vi "EditUser-Window.vi"(7 "Login-UI.lvlib:PwdMgr.lvclass":refnum<class "PwdMgr.lvclass">, 8 "error in":errorcluster, 9 "权  限":T1, 10 "密  码":string, 11 "用户名":string) -> (0 "error out":errorcluster)   [LabVIEW 2020, in "Login-UI.lvlib"]
uses:
  Login-UI.lvlib
  _Typedef/User-Role.ctl
  PwdMgr/PwdMgr.lvclass
  _Typedef/User-Info.ctl
panel:
  in  "Exit":bool
  in  "Save":bool
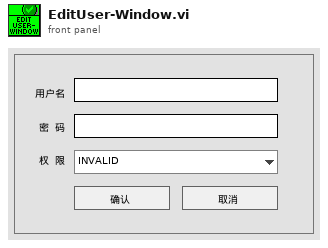
[diagram p1: front panel]
types:
  T1 = typedef "Login-UI.lvlib/User-Role.ctl" = enum16{"INVALID", "Operator", "Engineer", "Admin", "Anonymous"}
  T2 = enum32{"Invalid", "Standard", "Closed", "Hidden", "Minimized", "Maximized"}
  T3 = enum32{"invalid app kind", "Development System", "Run Time System", "Student Edition", "Embedded LabVIEW", "Evaluation", "Custom"}
  T4 = typedef "Login-UI.lvlib/User-Info.ctl" = cluster{"UserName":string, "Password":string, "Role":T1}
  T5 = cluster{"Core":cluster{"Current VI Reference":refnum<vi>, "Close Panel on Exit?":bool}, "Your Boolean data":bool, "Your string data":string, "Cluster":T4}
  T6 = typedef "eventvkey.ctl" = enum16{"ASCII", "Enter", "Return", "Shift", "Ctrl", "Alt", "Cmd", "Opt", "Caps", "NumLock", "Clear", "Break", "Up", "Down", "Left", "Right", "Insert", "Delete", "Home", "End", "PageUp", "PageDown", "Escape", "Help", "Pause", "ScrollLock", "F1", "F2", "F3", "F4", "F5", "F6", "F7", "F8", "F9", "F10", "F11", "F12", "F13", "F14", "F15", "F16", "F17", "F18", "F19", "F20", "F21", "F22", "F23", "F24", "Play", "VolumeUp", "VolumeDown", "Mute", "Two Byte Char"}
  T7 = cluster{"Current VI Reference":refnum<vi>, "Close Panel on Exit?":bool}
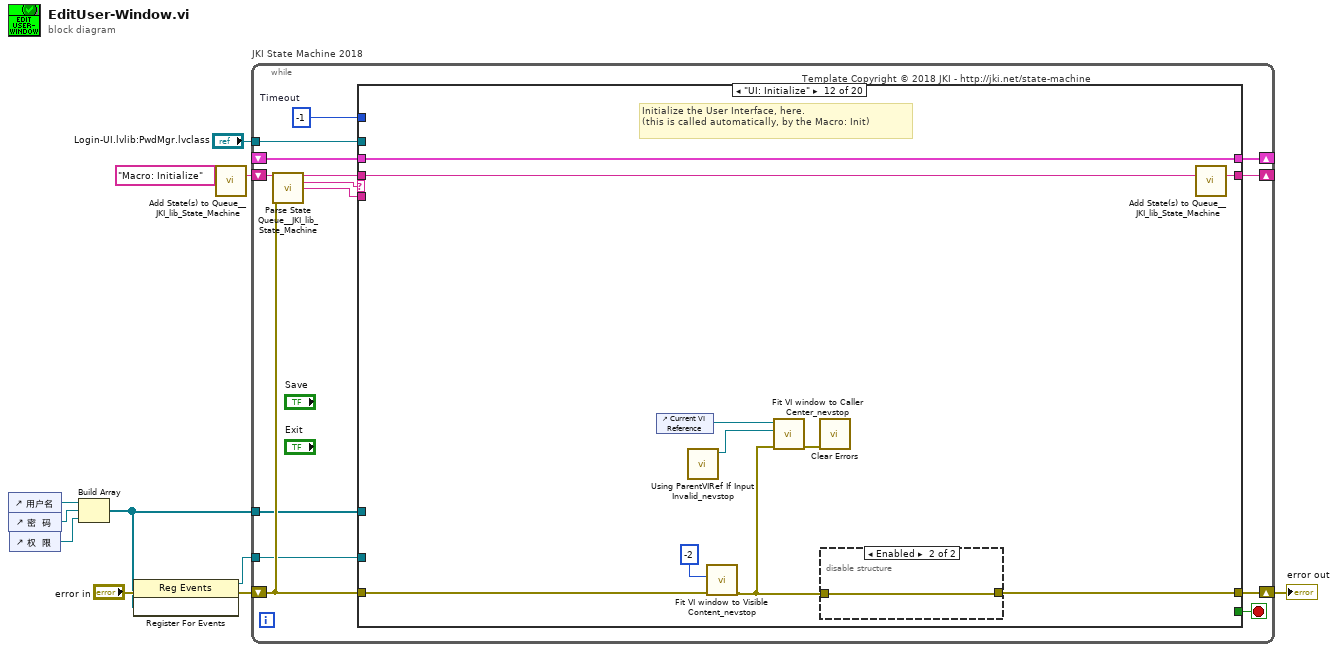
[diagram p0: block diagram]
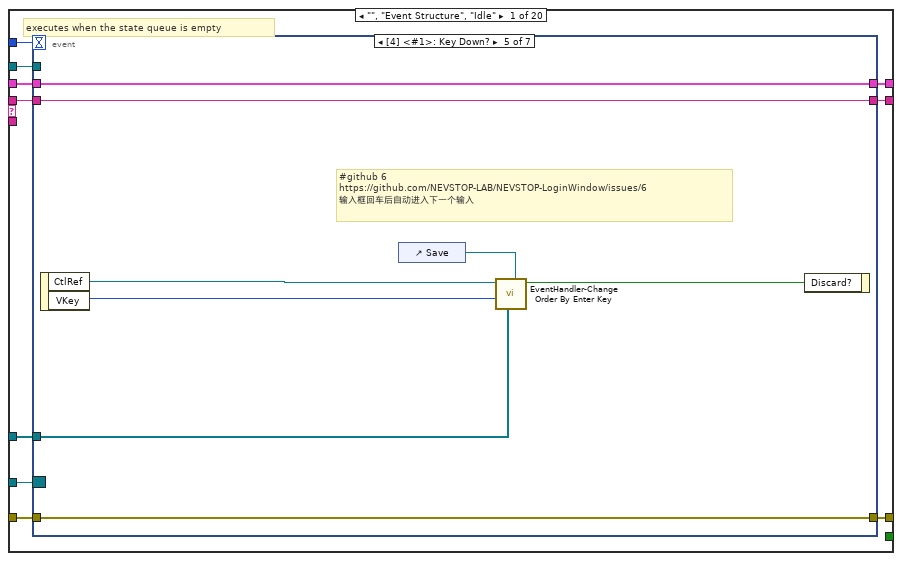
[diagram p2: hidden frame]
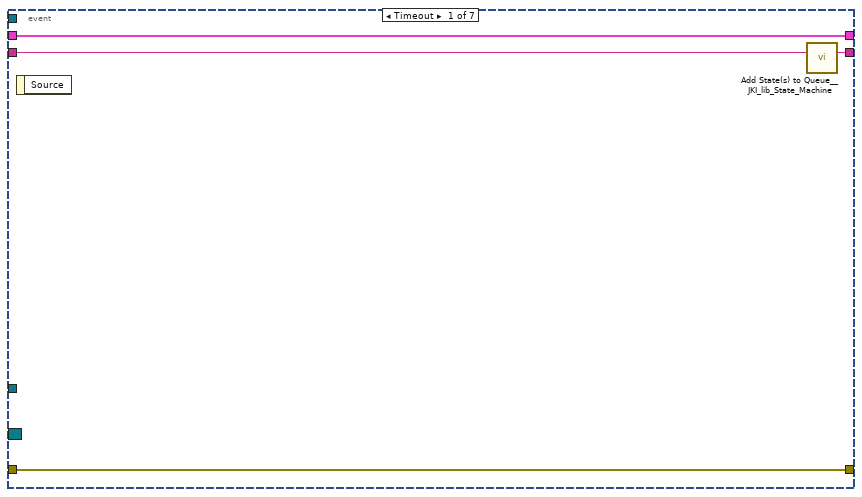
[diagram p3: hidden frame]
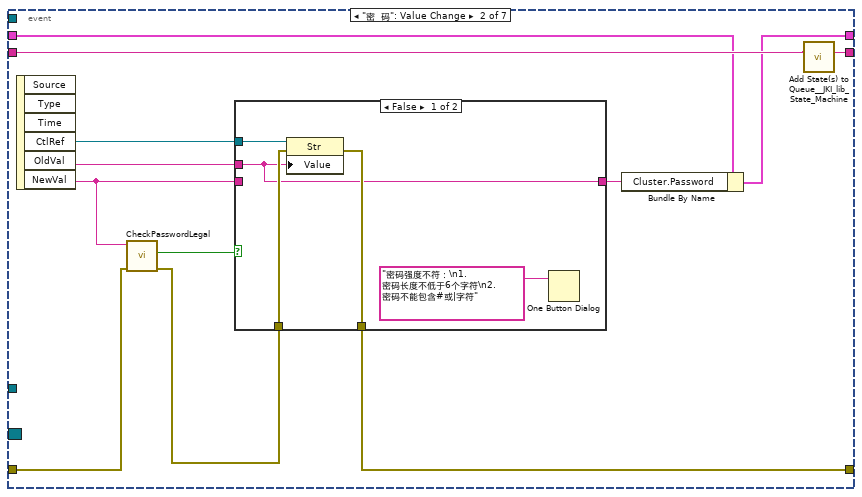
[diagram p4: hidden frame]
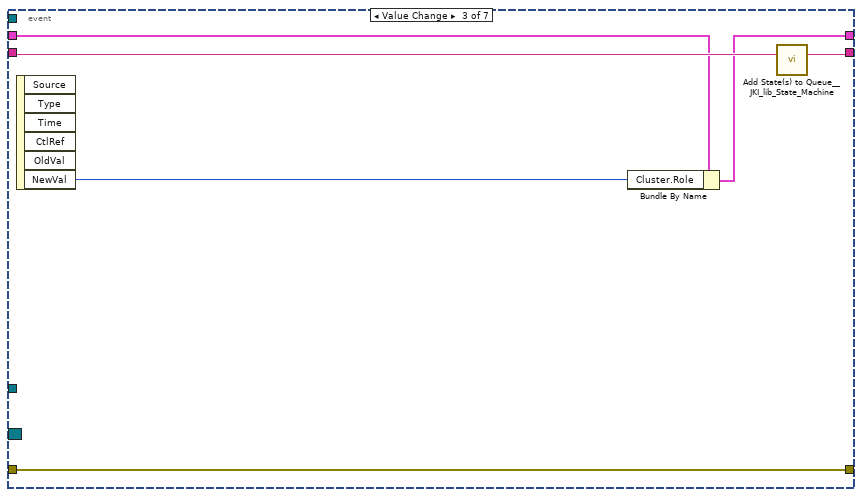
[diagram p6: hidden frame]
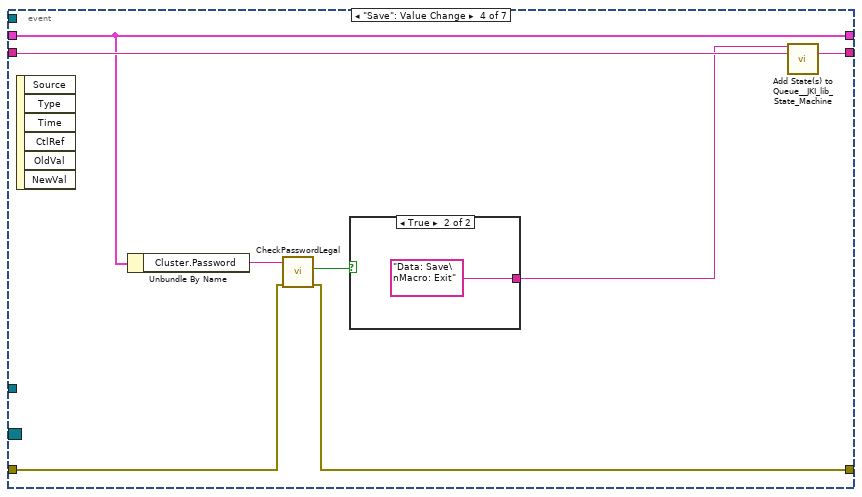
[diagram p7: hidden frame]
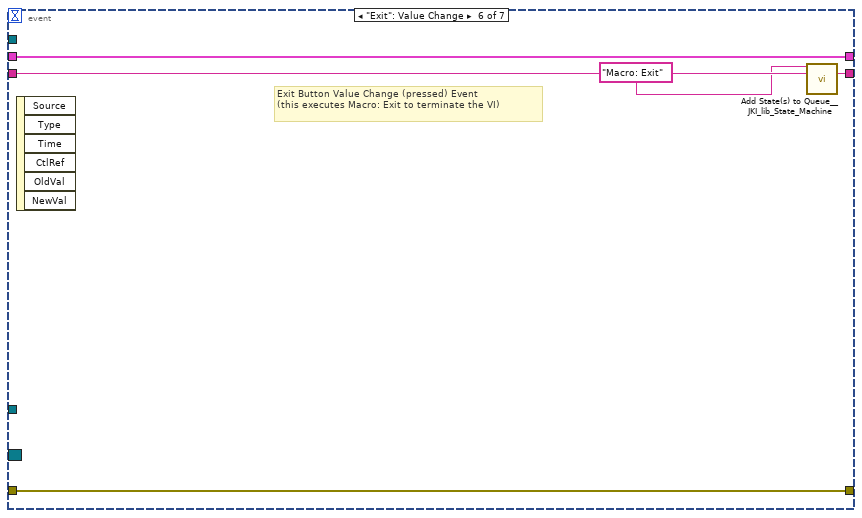
[diagram p9: hidden frame]
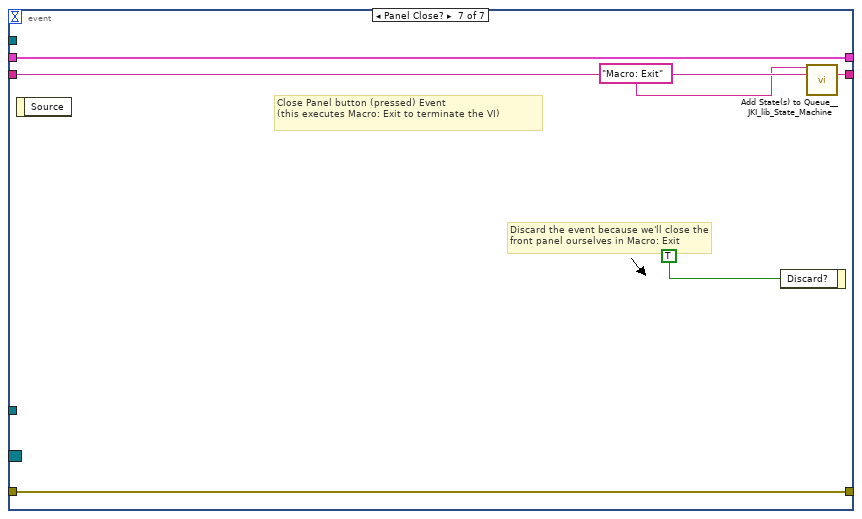
[diagram p10: hidden frame]
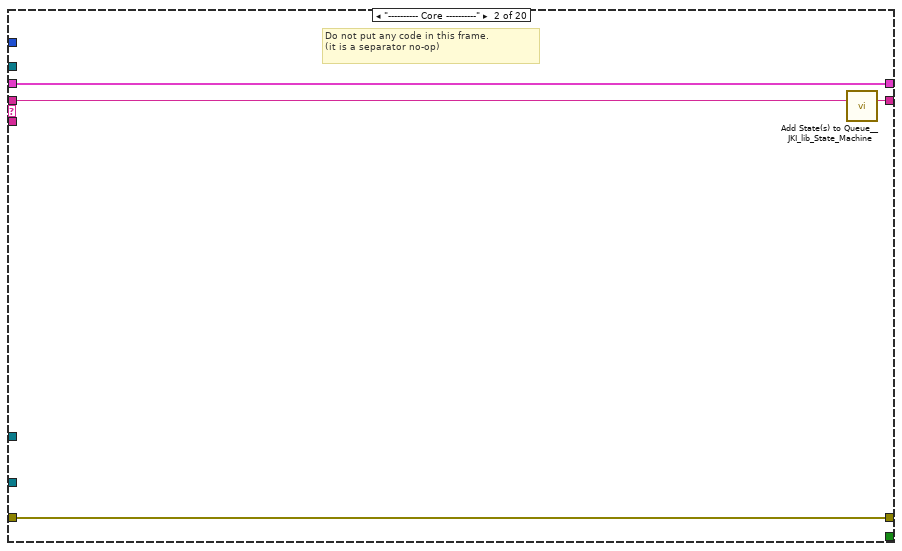
[diagram p11: hidden frame]
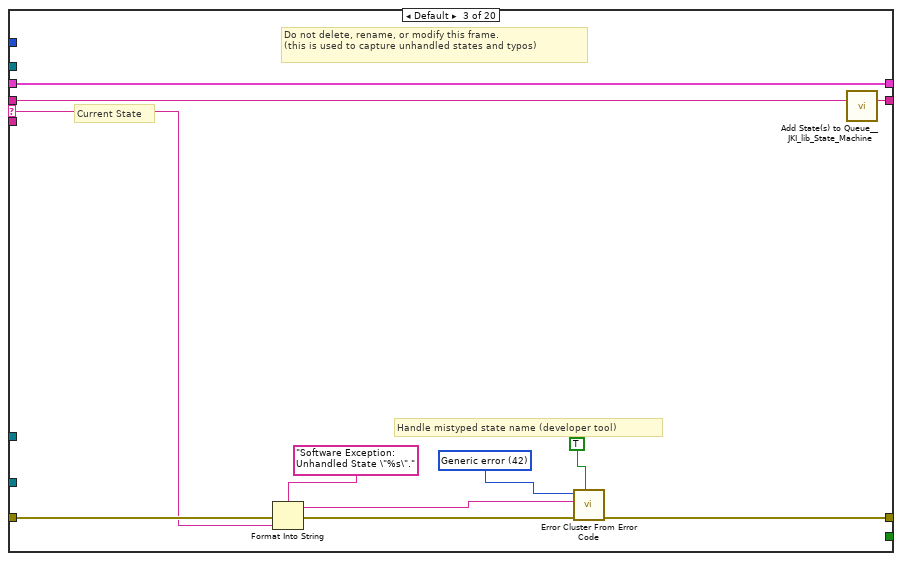
[diagram p12: hidden frame]
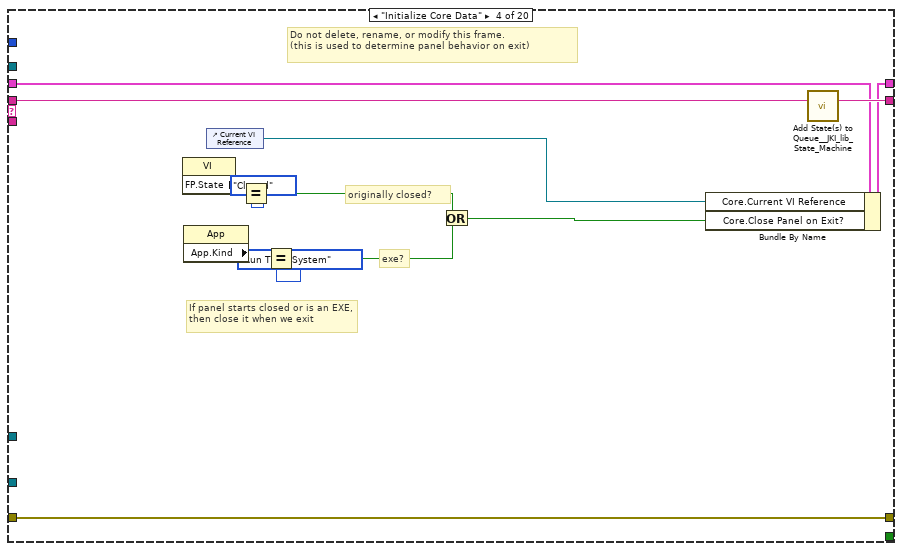
[diagram p13: hidden frame]
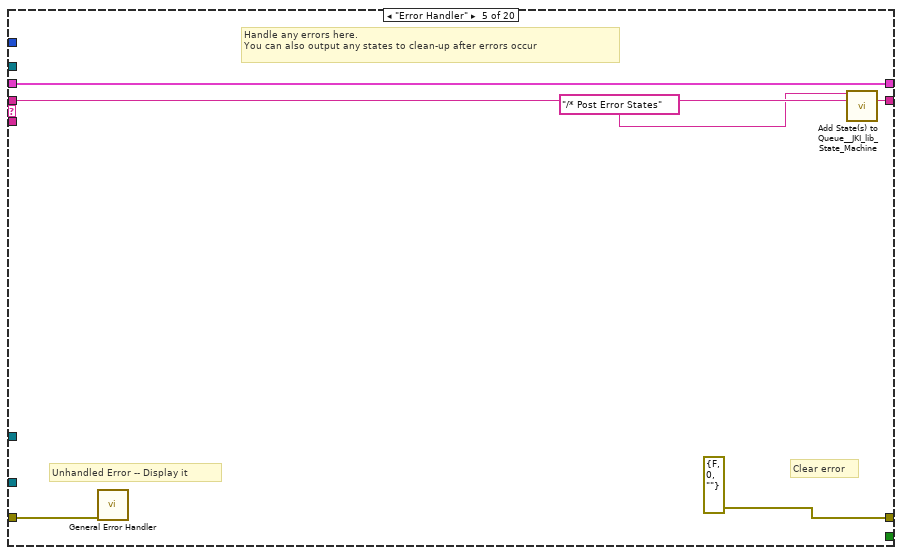
[diagram p14: hidden frame]
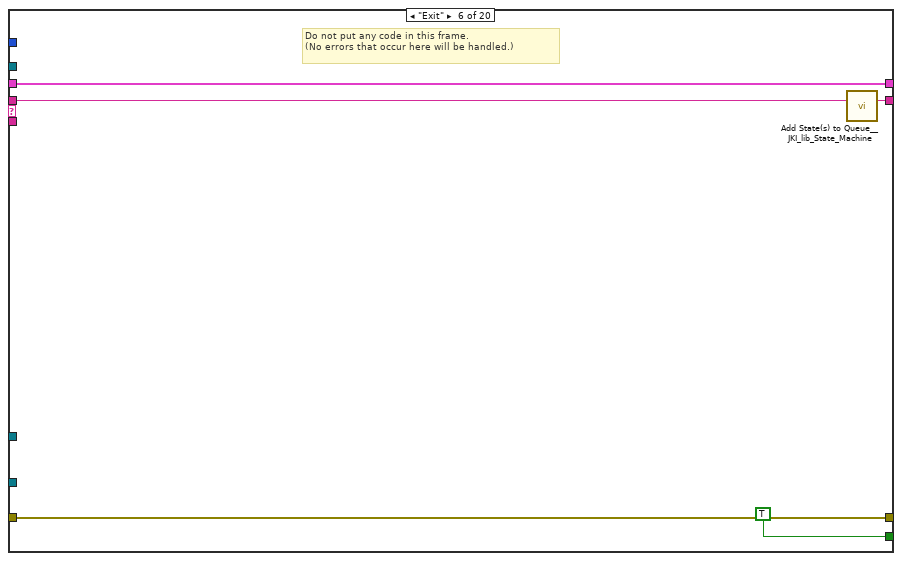
[diagram p15: hidden frame]
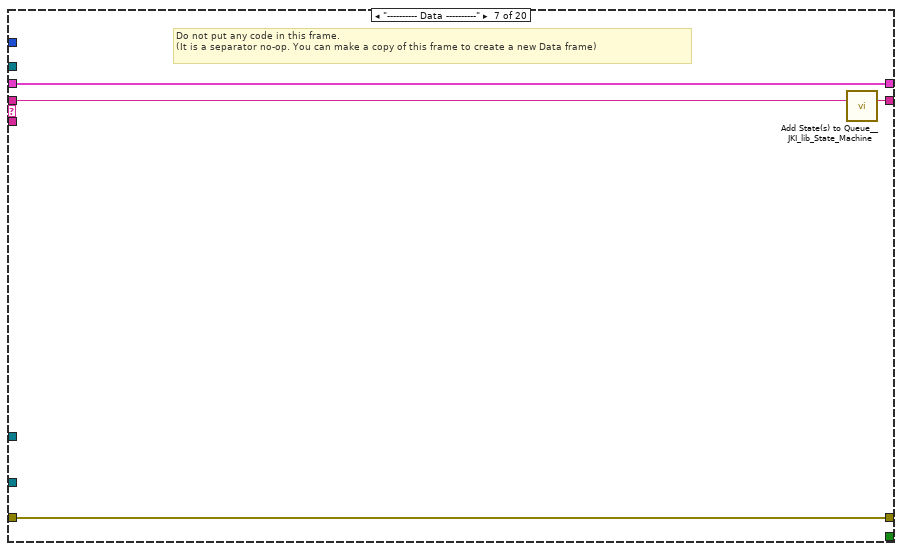
[diagram p16: hidden frame]
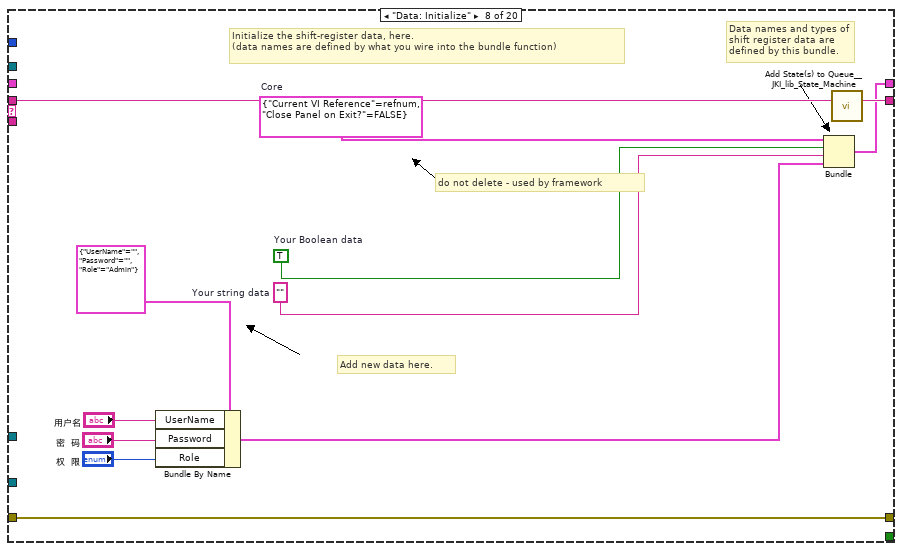
[diagram p17: hidden frame]
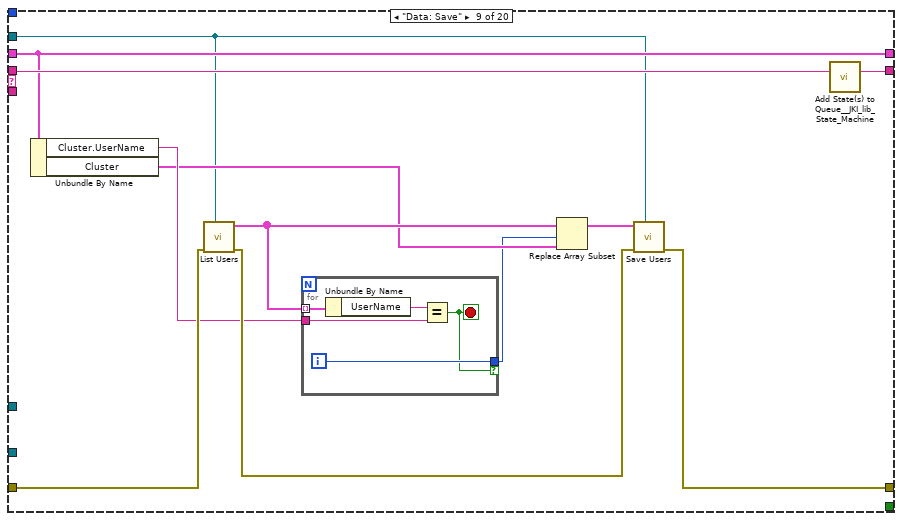
[diagram p18: hidden frame]
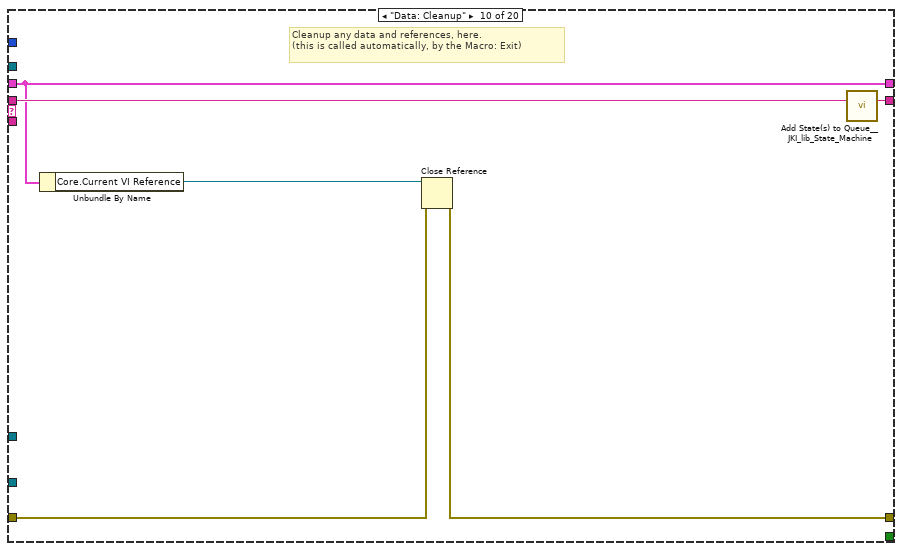
[diagram p19: hidden frame]
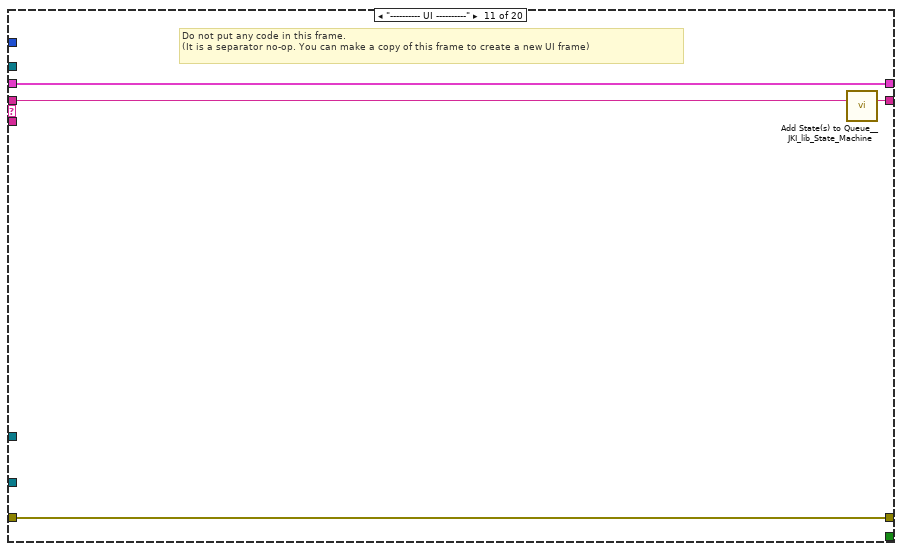
[diagram p20: hidden frame]
diagram:
  n1 = control-ref of="用户名"() -> (w6:refnum<vi>)
  n2 = control-ref of="密  码"() -> (w5:refnum<vi>)
  n3 = control-ref of="权  限"() -> (w4:refnum<vi>)
  n4 = Build Array(w6, w5, w4) -> (w2:refnum<vi>[])
  n5 = register-events(error in="error in", w2) -> (reference out=w3:refnum<event-registration>, error out=w7:errorcluster)  [unwired: 1 in]
  n6 = call <vilib>:"Add State(s) to Queue__JKI_lib_State_Machine.vi"("State(s) in (\"\")"="Macro: Initialize") -> ("States Out"=w11:string)  [unwired: 14 in]
  n7 = while "JKI State Machine 2018" {
    shift-right: [w18] -> _
    shift-left: _ -> [w17]
    shift-right: [w21] -> w8
    shift-left: w7 -> [w15]
    shift-right: [w20] -> _
    shift-left: w11 -> [w22]
    tunnel: w3 -> [w14]
    tunnel: w2 -> [w13]
    tunnel: "Login-UI.lvlib:PwdMgr.lvclass" -> [w12]
    stop <- w19 stop-if-true
    w16 = -1  # Timeout
    # "Template Copyright © 2018 JKI - http://jki.net/state-machine"
    n8 = call <vilib>:"Parse State Queue__JKI_lib_State_Machine.vi"("State Queue"=w22, "Error In (no error)"=w15) -> ("Remaining States"=w24:string, "Current State"=w25:string, "Arguments"=w23:string)  [unwired: 11 in]
    n9 = case shown="\"UI: Initialize\"" w25 {
      selector: w25 -> [_ _ w97 _ _ _ _ _ _ _ _ _ _ _ _ _ _ _ _ _]
      tunnel: w24 -> [w35 w96 w101 w120 w126 w131 w135 w147 w158 w170 w174 w184 w193 w204 w273 w278 w288 w292 w296 w300]
      tunnel: w23 -> [_ _ _ _ _ _ _ _ _ _ _ _ w188 w198 _ _ _ _ _ _]
      tunnel: w17 -> [w34 w93 w99 w113 w123 w129 w132 _ w157 w165 w171 w182 w191 w200 w270 w275 w285 w289 w293 w297]
      tunnel: [w33 w94 w103 w117 errorcluster {"status"=FALSE, "code"=0, "source"=""} ("error out") w128 w133 w144 w155 w166 w172 w179 w189 w201 w271 w276 w286 w290 w294 w298] -> w21
      tunnel: w15 -> [w32 w94 w102 w117 w122 w128 w133 w144 w156 w167 w172 w180 w190 w202 w271 w276 w286 w290 w294 w298]
      tunnel: [w29 w95 w100 w119 w125 w130 w134 w146 w159 w169 w173 w183 w192 w203 w272 w277 w287 w291 w295 w299] -> w20
      tunnel: [_ _ _ _ _ TRUE _ _ _ _ _ _ _ _ _ _ _ _ _ _] -> w19
      tunnel: [w31 w93 w99 w118 w123 w129 w132 w145 w157 w165 w171 w182 w191 w200 w270 w275 w285 w289 w293 w297] -> w18
      tunnel: w16 -> [w30 _ _ _ _ _ _ _ _ _ _ _ _ _ _ _ _ _ _ _]
      tunnel: w14 -> [w28 _ _ _ _ _ _ _ _ _ _ _ _ _ _ _ _ _ _ _]
      tunnel: w13 -> [w27 _ _ _ _ _ _ _ _ _ _ _ _ _ _ _ _ _ _ _]
      tunnel: w12 -> [w26 _ _ _ _ _ _ _ w148 _ _ _ _ _ _ _ _ _ _ _]
      frame "", "Event Structure", "Idle" {
        # "executes when the state queue is empty"
        n10 = event shown="[4] <#1>: Key Down?" {
          selector: w28 -> [_ _ _ _ _ _ _]
          dyn-events: _ -> [_ _ _ _ _ _ _]
          timeout: w30 -> [_ _ _ _ _ _ _]
          tunnel: w35 -> [w39 w47 w62 w71 w75 w86 w92]
          tunnel: [w38 w48 w63 w72 w75 w85 w91] -> w29
          tunnel: w34 -> [w36 w42 w61 w69 w76 w83 w89]
          tunnel: [w37 w49 w64 w65 w81 w84 w90] -> w33
          tunnel: w32 -> [w37 w45 w64 w66 w81 w84 w90]
          tunnel: [w36 w40 w60 w69 w76 w83 w89] -> w31
          tunnel: w27 -> [_ _ _ _ w78 _ _]
          tunnel: w26 -> [_ _ _ _ _ _ _]
          event Timeout {
            n11 = event-data() -> ()  [unwired: 1 in, 1 out]
            n12 = call <vilib>:"Add State(s) to Queue__JKI_lib_State_Machine.vi"("State(s) in (\"\")"=w39) -> ("States Out"=w38:string)  [unwired: 14 in]
          }
          event "密  码": Value Change {
            n13 = event-data() -> ("CtlRef"=w50:refnum<vi>, "OldVal"=w51:string, "NewVal"=w46:string)  [unwired: 1 in, 3 out]
            n14 = call "CheckPasswordLegal.vi"("error in (no error)"=w45, "Password"=w46) -> ("error out"=w44:errorcluster, "legal?"=w43:bool)  [unwired: 8 in]
            n15 = case shown="False" w43 {
              tunnel: w51 -> [w52 _]
              tunnel: w46 -> [_ w57]
              tunnel: [w55 w58] -> w49
              tunnel: w50 -> [w54 _]
              tunnel: w44 -> [w53 w58]
              tunnel: [w52 w57] -> w41
              frame False {
                n16 = property class="Str"(reference=w54, error in=w53, "Value"=w52) -> (error out=w55:errorcluster)  [unwired: 1 out]
                n17 = One Button Dialog(message="密码强度不符：\n1.密码长度不低于6个字符\n2. 密码不能包含#或|字符") -> ()  [unwired: 1 in, 1 out]
              }
              frame True {
              }
            }
            n18 = Bundle By Name(cluster=w42, "Cluster.Password"=w41) -> (w40:T5)
            n19 = call <vilib>:"Add State(s) to Queue__JKI_lib_State_Machine.vi"("State(s) in (\"\")"=w47) -> ("States Out"=w48:string)  [unwired: 14 in]
          }
          event Value Change {
            n20 = event-data() -> ("NewVal"=w59:T1)  [unwired: 1 in, 5 out]
            n21 = Bundle By Name(cluster=w61, "Cluster.Role"=w59) -> (w60:T5)
            n22 = call <vilib>:"Add State(s) to Queue__JKI_lib_State_Machine.vi"("State(s) in (\"\")"=w62) -> ("States Out"=w63:string)  [unwired: 14 in]
          }
          event "Save": Value Change {
            n23 = event-data() -> ()  [unwired: 1 in, 6 out]
            n24 = Unbundle By Name(w69) -> ("Cluster.Password"=w70:string)
            n25 = call "CheckPasswordLegal.vi"("error in (no error)"=w66, "Password"=w70) -> ("error out"=w65:errorcluster, "legal?"=w67:bool)  [unwired: 8 in]
            n26 = case shown="True" w67 {
              tunnel: [_ "Data: Save\nMacro: Exit"] -> w68
              frame False {
              }
              frame True {
              }
            }
            n27 = call <vilib>:"Add State(s) to Queue__JKI_lib_State_Machine.vi"("State(s) in Front (\"\")"=w68, "State(s) in (\"\")"=w71) -> ("States Out"=w72:string)  [unwired: 13 in]
          }
          event Key Down? {
            # "#github 6\nhttps://github.com/NEVSTOP-LAB/NEVSTOP-LoginWindow/issues/6\n输入框回车后自动进入下一个输入"
            n28 = event-data() -> ("CtlRef"=w80:refnum<vi>, "VKey"=w79:T6)  [unwired: 1 in]
            n29 = control-ref of="Save"() -> (w74:refnum<vi>)
            n30 = call "EventHandler-Change Order By Enter Key.vi"("Next Ctrl"=w74, "Controls for changing order"=w78, "VKey"=w79, "Event Control"=w80) -> ("Discard?"=w77:bool)  [unwired: 7 in]
            n31 = event-data("Discard?"=w77) -> ()  [unwired: 1 in, 1 out]
          }
          event "Exit": Value Change {
            # "Exit Button Value Change (pressed) Event\n(this executes Macro: Exit to terminate the VI)"
            n32 = event-data() -> ()  [unwired: 1 in, 6 out]
            n33 = call <vilib>:"Add State(s) to Queue__JKI_lib_State_Machine.vi"("State(s) in Front (\"\")"="Macro: Exit", "State(s) in (\"\")"=w86) -> ("States Out"=w85:string)  [unwired: 13 in]
          }
          event Panel Close? {
            # "Discard the event because we'll close the front panel ourselves in Macro: Exit"
            # "Close Panel button (pressed) Event\n(this executes Macro: Exit to terminate the VI)"
            n34 = event-data() -> ()  [unwired: 1 in, 1 out]
            n35 = event-data("Discard?"=TRUE) -> ()  [unwired: 1 in, 1 out]
            n36 = call <vilib>:"Add State(s) to Queue__JKI_lib_State_Machine.vi"("State(s) in Front (\"\")"="Macro: Exit", "State(s) in (\"\")"=w92) -> ("States Out"=w91:string)  [unwired: 13 in]
          }
        }
      }
      frame "---------- Core ----------" {
        # "Do not put any code in this frame.\n(it is a separator no-op)"
        n37 = call <vilib>:"Add State(s) to Queue__JKI_lib_State_Machine.vi"("State(s) in (\"\")"=w96) -> ("States Out"=w95:string)  [unwired: 14 in]
      }
      frame Default {
        w106 = 42 items=["No error", "Argument error", "Memory is full", "Out of zone", "End of file", "File already open", "Generic file I/O error", "File not found", "File permission error", "Disk is full", "Duplicate path", "Too many files open", "System feature not enabled", "Resource file not found", "Cannot add resource", "Resource not found", "Image not found", "Image memory error", "Pen does not exist", "Config type invalid", "Config token not found", "Config parse error", "Config memory error", "Bad external code format", "Bad external code offset", "External code not present", "Null window", "Destroy window error", "Null menu", "Print aborted", "Bad print record", "Print driver error", "Windows error during printing", "Memory error during printing", "Print dialog error", "Generic print error", "Invalid device refnum", "Device not found", "Device parameter error", "Device unit error", "Cannot open device", "Device call aborted", "Generic error", "Cancelled by user", "Object ID too low", "Object ID too high", "Object not in heap", "Unknown heap", "Unknown object (invalid DefProc)", "Unknown object (DefProc not in table)", "Message out of range", "Invalid (null) method", "Unknown message", "Manager call not supported", "Bad address", "Network operation in progress", "Network operation timed out", "Connection is busy", "Network attribute not supported", "Network error", "Address in use", "System out of memory", "Connection aborted", "Connection refused", "Not connected", "Already connected", "Connection closed", "Initialization error (interapplication manager)", "Bad occurrence", "Wait on unbound occurrence handler", "Occurrence queue overflow", "Datalog type conflict", "Unused", "Unrecognized type (interapplication manager)", "Memory corrupt", "Failed to make temporary DLL", "Old CIN version", "Drag socket not found", "Failed to load drop-object", "Failed to register OLE object", "Failed to release OLE object", "Format specifier type mismatch", "Unknown format specifier", "Too few format specifiers", "Too many format specifiers", "Scan failed", "Newer CIN version", "Error converting to variant", "Runtime menu error", "Password tampered", "Variant attribute not found", "Incompatible variant data type", "Event data is not available", "Event Store is not present", "Occurrence is not found", "Event Queue is not created", "Event info is not available", "Refnum passed is NULL", "Error retrieving Class GUID", "Error retrieving CoClass GUID", "Error retrieving TypeLib GUID.", "Bad built application magic bytes.", "Specific driver is different from the specific driver associated with the Logical Name.", "There is no session opened to the class driver.", "Max Error", "MAX - Error with config objects", "MAX - Error loading configuration", "MAX - Group not supported"]
        # "Current State"
        # "Do not delete, rename, or modify this frame.\n(this is used to capture unhandled states and typos)"
        # "Handle mistyped state name (developer tool)"
        n38 = Format Into String(format string="Software Exception: Unhandled State \"%s\"." ("message"), error in=w102, w97) -> (resulting string=w105:string, error out=w104:errorcluster)  [unwired: 1 in]
        n39 = call <vilib>:"Error Cluster From Error Code.vi"("show call chain? (False)"=TRUE, "error in (no error)"=w104, "error message (\"\")"=w105, "error code (0)"=w106) -> ("error out"=w103:errorcluster)  [unwired: 5 in]
        n40 = call <vilib>:"Add State(s) to Queue__JKI_lib_State_Machine.vi"("State(s) in (\"\")"=w101) -> ("States Out"=w100:string)  [unwired: 14 in]
      }
      frame "Initialize Core Data" {
        # "Do not delete, rename, or modify this frame.\n(this is used to determine panel behavior on exit)"
        # "originally closed?"
        # "exe?"
        # "If panel starts closed or is an EXE, then close it when we exit"
        n41 = property class="VI"() -> ("FP.State"=w110:T2)  [unwired: 2 in, 2 out]
        n42 = property class="App"() -> ("App.Kind"=w116:T3)  [unwired: 2 in, 2 out]
        n43 = control-ref of="Current VI Reference"() -> (w111:refnum<vi>)
        n44 = Equal?(x=w110, y=T2."Closed" ("Front Panel Window:State")) -> (x = y?=w108:bool)
        n45 = Equal?(x=w116, y=T3."Run Time System" ("Application:Kind")) -> (x = y?=w114:bool)
        n46 = Or(x=w108, y=w114) -> (x .or. y?=w112:bool)
        n47 = Bundle By Name(cluster=w113, "Core.Current VI Reference"=w111, "Core.Close Panel on Exit?"=w112) -> (w118:T5)
        n48 = call <vilib>:"Add State(s) to Queue__JKI_lib_State_Machine.vi"("State(s) in (\"\")"=w120) -> ("States Out"=w119:string)  [unwired: 14 in]
      }
      frame "Error Handler" {
        # "Unhandled Error -- Display it"
        # "Handle any errors here.\nYou can also output any states to clean-up after errors occur"
        # "Clear error"
        n49 = call <vilib>:"General Error Handler.vi"("error in (no error)"=w122) -> ()  [unwired: 10 in, 5 out]
        n50 = call <vilib>:"Add State(s) to Queue__JKI_lib_State_Machine.vi"("State(s) in Front (\"\")"="/* Post Error States", "State(s) in (\"\")"=w126) -> ("States Out"=w125:string)  [unwired: 13 in]
      }
      frame "Exit" {
        # "Do not put any code in this frame.\n(No errors that occur here will be handled.)"
        n51 = call <vilib>:"Add State(s) to Queue__JKI_lib_State_Machine.vi"("State(s) in (\"\")"=w131) -> ("States Out"=w130:string)  [unwired: 14 in]
      }
      frame "---------- Data ----------" {
        # "Do not put any code in this frame.\n(It is a separator no-op. You can make a copy of this frame to create a new Data frame)"
        n52 = call <vilib>:"Add State(s) to Queue__JKI_lib_State_Machine.vi"("State(s) in (\"\")"=w135) -> ("States Out"=w134:string)  [unwired: 14 in]
      }
      frame "Data: Initialize" {
        w141 = T7 {"Current VI Reference"=refnum, "Close Panel on Exit?"=FALSE}  # Core
        w143 = TRUE  # Your Boolean data
        w142 = ""  # Your string data
        # "do not delete - used by framework"
        # "Add new data here."
        # "Data names and types of shift register data are defined by this bundle."
        # "Initialize the shift-register data, here.\n(data names are defined by what you wire into the bundle function)"
        n53 = Bundle By Name(cluster=T4 {"UserName"="", "Password"="", "Role"=enum."Admin"} ("Cluster"), "UserName"="用户名", "Password"="密  码", "Role"="权  限") -> (w136:T4)
        n54 = Bundle("Core"=w141, "Your Boolean data"=w143, "Your string data"=w142, "Cluster"=w136) -> (w145:T5)  [unwired: 1 in]
        n55 = call <vilib>:"Add State(s) to Queue__JKI_lib_State_Machine.vi"("State(s) in (\"\")"=w147) -> ("States Out"=w146:string)  [unwired: 14 in]
      }
      frame "Data: Save" {
        n56 = Unbundle By Name(w157) -> ("Cluster.UserName"=w153:string, "Cluster"=w151:T4)
        n57 = call-dynamic "List Users.vi"("PwdMgr in"=w148, "error in (no error)"=w156) -> ("error out"=w154:errorcluster, "Array"=w152:T4[])  [unwired: 8 in]
        n58 = for {
          tunnel: w152 -> [w164] mode=indexing
          tunnel: w153 -> [w162]
          tunnel: [w161] -> w150 if=w160
          i -> [w161]
          stop <- w160 stop-if-true
          n59 = Unbundle By Name(w164) -> ("UserName"=w163:string)
          n60 = Equal?(x=w163, y=w162) -> (x = y?=w160:bool)
        }
        n61 = Replace Array Subset(array=w152, new element=w151, index=w150) -> (w149:T4[])
        n62 = call-dynamic "Save Users.vi"("PwdMgr in"=w148, "error in (no error)"=w154, "Array"=w149) -> ("error out"=w155:errorcluster)  [unwired: 8 in]
        n63 = call <vilib>:"Add State(s) to Queue__JKI_lib_State_Machine.vi"("State(s) in (\"\")"=w158) -> ("States Out"=w159:string)  [unwired: 14 in]
      }
      frame "Data: Cleanup" {
        # "Cleanup any data and references, here.\n(this is called automatically, by the Macro: Exit)"
        n64 = Unbundle By Name(w165) -> ("Core.Current VI Reference"=w168:refnum<vi>)
        n65 = Close Reference(reference=w168, error in (no error)=w167) -> (error out=w166:errorcluster)
        n66 = call <vilib>:"Add State(s) to Queue__JKI_lib_State_Machine.vi"("State(s) in (\"\")"=w170) -> ("States Out"=w169:string)  [unwired: 14 in]
      }
      frame "---------- UI ----------" {
        # "Do not put any code in this frame.\n(It is a separator no-op. You can make a copy of this frame to create a new UI frame)"
        n67 = call <vilib>:"Add State(s) to Queue__JKI_lib_State_Machine.vi"("State(s) in (\"\")"=w174) -> ("States Out"=w173:string)  [unwired: 14 in]
      }
      frame "UI: Initialize" {
        # "Initialize the User Interface, here.\n(this is called automatically, by the Macro: Init)"
        n68 = control-ref of="Current VI Reference"() -> (w177:refnum<vi>)
        n69 = call <userlib>:"Using ParentVIRef If Input Invalid_nevstop.vi"() -> ("VI Ref"=w176:refnum<vi>)  [unwired: 6 in, 1 out]
        n70 = call <userlib>:"Fit VI window to Visible Content_nevstop.vi"("error in (no error)"=w180, "border spacing (2 px)"=-2) -> ("error out"=w175:errorcluster)  [unwired: 4 in, 1 out]
        n71 = call <userlib>:"Fit VI window to Caller Center_nevstop.vi"("Error In"=w175, "Background VI Ref (Callee's Caller)"=w176, "VI Ref (calling VI)"=w177) -> ("Error Out"=w178:errorcluster)  [unwired: 3 in, 1 out]
        n72 = call <vilib>:"Clear Errors.vi"("error in (no error)"=w178) -> ()  [unwired: 5 in, 2 out]
        n73 = disable-structure shown="Enabled" {
          disable-tunnel: w175 -> [w186 w187]
          disable-tunnel: [w185 w187] -> w179
          frame Disabled {
            n74 = invoke class="VI" method="Default Vals.Reinit All"(error in=w186) -> (error out=w185:errorcluster)  [unwired: 2 in, 2 out]
          }
          frame Enabled {
          }
        }
        n75 = call <vilib>:"Add State(s) to Queue__JKI_lib_State_Machine.vi"("State(s) in (\"\")"=w184) -> ("States Out"=w183:string)  [unwired: 14 in]
      }
      frame "UI: Cursor Set" {
        # "Argument"
        # "Set and Unset Cursor Busy.\n(Usage: \"UI: Cursor Set >> Busy|Idle\")"
        n76 = case shown="\"Idle\", Default" w188 {
          tunnel: w190 -> [w195 w197]
          tunnel: [w194 w196] -> w189
          frame "Idle", Default {
            n77 = call <vilib>:"Unset Busy.vi"("error in (no error)"=w195) -> ("error out"=w194:errorcluster)  [unwired: 10 in]
          }
          frame "Busy" {
            n78 = call <vilib>:"Set Busy.vi"("error in (no error)"=w197) -> ("error out"=w196:errorcluster)  [unwired: 9 in, 1 out]
          }
        }
        n79 = call <vilib>:"Add State(s) to Queue__JKI_lib_State_Machine.vi"("State(s) in (\"\")"=w193) -> ("States Out"=w192:string)  [unwired: 14 in]
      }
      frame "UI: Front Panel State" {
        # "Argument"
        # "Set Front Panel Open or Closed\n(Usage: \"UI: Front Panel State >> Open|Close\")"
        n80 = Unbundle By Name(w200) -> ("Core.Current VI Reference"=w199:refnum<vi>)
        n81 = case shown="\"Minimize\", \"Minimized\"" w198 {
          tunnel: w202 -> [w210 w225 w236 w249 w262]
          tunnel: [w212 w226 w238 w251 w264] -> w201
          tunnel: w199 -> [w211 w223 w237 w250 w263]
          frame "Open", "Standard", Default {
            w205 = T2."Standard" ("State")
            n82 = property class="VI"(reference=w211, error in=w210) -> (reference out=w208:refnum<vi>, error out=w209:errorcluster, "FP.State"=w207:T2)
            n83 = Not Equal?(x=w207, y=w205) -> (x != y?=w206:bool)
            n84 = case shown="True" w206 {
              tunnel: [w216 w218] -> w212
              tunnel: w209 -> [w215 w218]
              tunnel: w208 -> [w214 _]
              tunnel: w205 -> [w213 _]
              frame True {
                n85 = invoke class="VI" method="FP.Open"(reference=w214, error in=w215, "Activate"=TRUE, "State"=w213) -> (error out=w216:errorcluster)  [unwired: 1 in, 4 out]
              }
              frame False {
              }
            }
          }
          frame "Close", "Closed" {
            n86 = property class="VI"(reference=w223, error in=w225) -> (reference out=w222:refnum<vi>, error out=w224:errorcluster, "FP.State"=w220:T2)
            n87 = Not Equal?(x=w220, y=T2."Closed" ("Front Panel Window:State")) -> (x != y?=w219:bool)
            n88 = case shown="True" w219 {
              tunnel: [w227 w230] -> w226
              tunnel: w224 -> [w227 w229]
              tunnel: w222 -> [_ w228]
              frame False {
              }
              frame True {
                n89 = invoke class="VI" method="FP.Close"(reference=w228, error in=w229) -> (error out=w230:errorcluster)  [unwired: 1 in, 2 out]
              }
            }
          }
          frame "Hidden", "Hide" {
            w231 = T2."Hidden" ("State")
            n90 = property class="VI"(reference=w237, error in=w236) -> (reference out=w234:refnum<vi>, error out=w235:errorcluster, "FP.State"=w233:T2)
            n91 = Not Equal?(x=w233, y=w231) -> (x != y?=w232:bool)
            n92 = case shown="True" w232 {
              tunnel: [w242 w243] -> w238
              tunnel: w235 -> [w241 w243]
              tunnel: w234 -> [w240 _]
              tunnel: w231 -> [w239 _]
              frame True {
                n93 = invoke class="VI" method="FP.Open"(reference=w240, error in=w241, "State"=w239) -> (error out=w242:errorcluster)  [unwired: 2 in, 4 out]
              }
              frame False {
              }
            }
          }
          frame "Minimize", "Minimized" {
            w244 = T2."Minimized" ("State")
            n94 = property class="VI"(reference=w250, error in=w249) -> (reference out=w247:refnum<vi>, error out=w248:errorcluster, "FP.State"=w246:T2)
            n95 = Not Equal?(x=w246, y=w244) -> (x != y?=w245:bool)
            n96 = case shown="True" w245 {
              tunnel: [w255 w256] -> w251
              tunnel: w248 -> [w254 w256]
              tunnel: w247 -> [w253 _]
              tunnel: w244 -> [w252 _]
              frame True {
                n97 = invoke class="VI" method="FP.Open"(reference=w253, error in=w254, "State"=w252) -> (error out=w255:errorcluster)  [unwired: 2 in, 4 out]
              }
              frame False {
              }
            }
          }
          frame "Maximize", "Maximized" {
            w257 = T2."Maximized" ("State")
            n98 = property class="VI"(reference=w263, error in=w262) -> (reference out=w260:refnum<vi>, error out=w261:errorcluster, "FP.State"=w259:T2)
            n99 = Not Equal?(x=w259, y=w257) -> (x != y?=w258:bool)
            n100 = case shown="True" w258 {
              tunnel: [w268 w269] -> w264
              tunnel: w261 -> [w267 w269]
              tunnel: w260 -> [w266 _]
              tunnel: w257 -> [w265 _]
              frame True {
                n101 = invoke class="VI" method="FP.Open"(reference=w266, error in=w267, "State"=w265) -> (error out=w268:errorcluster)  [unwired: 2 in, 4 out]
              }
              frame False {
              }
            }
          }
        }
        n102 = call <vilib>:"Add State(s) to Queue__JKI_lib_State_Machine.vi"("State(s) in (\"\")"=w204) -> ("States Out"=w203:string)  [unwired: 14 in]
      }
      frame "---------- Macro ----------" {
        # "Do not put any code in this frame.\n(It is a separator no-op. You can make a copy of this frame to create a new Macro frame)"
        n103 = call <vilib>:"Add State(s) to Queue__JKI_lib_State_Machine.vi"("State(s) in (\"\")"=w273) -> ("States Out"=w272:string)  [unwired: 14 in]
      }
      frame "Macro: Initialize" {
        w274 = "Data: Initialize\nInitialize Core Data\nUI: Initialize\nUI: Front Panel State >> Open"  # Data: Initialize Initialize Core Data UI: Initialize UI: Front Panel State >> Open
        # "Initialization Macro\n(This is called once, when the VI starts)"
        n104 = call <vilib>:"Add State(s) to Queue__JKI_lib_State_Machine.vi"("State(s) in Front (\"\")"=w274, "State(s) in (\"\")"=w278) -> ("States Out"=w277:string)  [unwired: 13 in]
      }
      frame "Macro: Exit" {
        # "Exit Macro\n(This is called once, when the VI exits)"
        n105 = Unbundle By Name(w285) -> ("Core.Close Panel on Exit?"=w284:bool)
        n106 = Select(t="UI: Front Panel State >> Close", s=w284, f="") -> (s? t:f=w281:string)
        n107 = call <vilib>:"Add State(s) to Queue__JKI_lib_State_Machine.vi"("State(s) in (\"\")"=w281, "State(s) at Back (\"\")"="Data: Cleanup\nExit") -> ("States Out"=w279:string)  [unwired: 13 in]
        n108 = call <vilib>:"Add State(s) to Queue__JKI_lib_State_Machine.vi"("State(s) in Front (\"\")"=w279, "State(s) in (\"\")"=w288) -> ("States Out"=w287:string)  [unwired: 13 in]
      }
      frame "---------- New Category ----------" {
        # "Template Separator\n(You can make a copy of, or modify, this frame)"
        n109 = call <vilib>:"Add State(s) to Queue__JKI_lib_State_Machine.vi"("State(s) in (\"\")"=w292) -> ("States Out"=w291:string)  [unwired: 14 in]
      }
      frame "New Category: 1" {
        # "Your code here.\n(You can make a copy of, or modify, this frame)"
        n110 = call <vilib>:"Add State(s) to Queue__JKI_lib_State_Machine.vi"("State(s) in (\"\")"=w296) -> ("States Out"=w295:string)  [unwired: 14 in]
      }
      frame "New Category: 2" {
        # "Your code here.\n(You can make a copy of, or modify, this frame)"
        n111 = call <vilib>:"Add State(s) to Queue__JKI_lib_State_Machine.vi"("State(s) in (\"\")"=w300) -> ("States Out"=w299:string)  [unwired: 14 in]
      }
    }
  }
  "error out" <- w8
